vi "Load Configuration Database.vi"(8 "error in (no error)":errorcluster, 10 "Configuration Database Type":T1, 11 "Simulated Configuration Database in":refnum<class "Simulated Configuration Database.lvclass">) -> (0 "error out":errorcluster, 3 "Simulated Configuration Database out":refnum<class "Simulated Configuration Database.lvclass">)   [LabVIEW 2012, in "Simulated Configuration Database.lvlib" / "Simulated Configuration Database.lvclass"]
uses:
  Simulated Configuration Database.lvclass
  Configuration Database API/Configuration Database API/Configuration Type.ctl
  Configuration Database API/Configuration Database API/Record.ctl
  Configuration Database API/Configuration Database API/Configuration Database API.lvclass
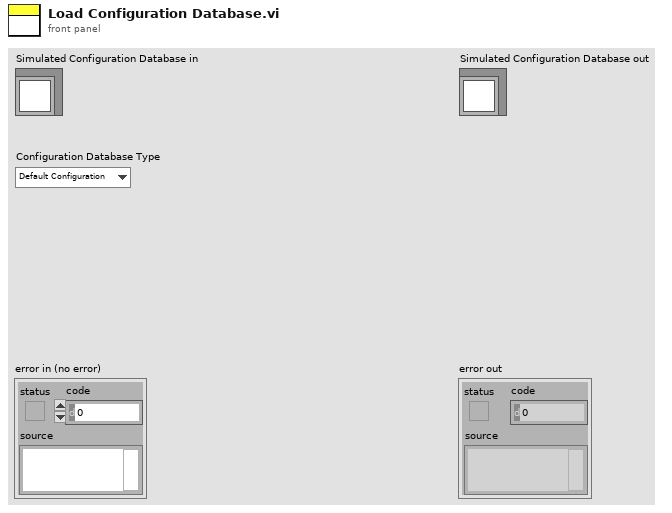
[diagram p1: front panel]
types:
  T1 = typedef "Configuration Database API.lvlib/Configuration Database API.lvclass/Configuration Type.ctl" = enum16{"Default Configuration", "Client Configuration"}
  T2 = typedef "Configuration Database API.lvlib/Configuration Database API.lvclass/Record.ctl" = cluster{"Wash Step":string, "Station":string, "Step Duration":u8}
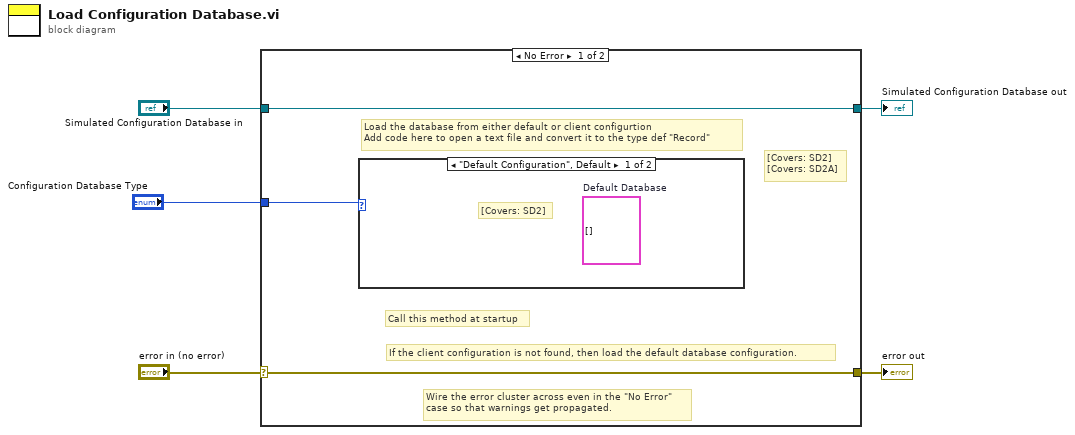
[diagram p0: block diagram]
diagram:
  n1 = case shown="No Error" "error in (no error)" {
    selector: "error in (no error)" -> [w7 w10]
    tunnel: [w7 w10] -> w4
    tunnel: [w8 w9] -> w2
    tunnel: "Simulated Configuration Database in" -> [w8 w9]
    tunnel: "Configuration Database Type" -> [w6 _]
    frame No Error {
      # "If the client configuration is not found, then load the default database configuration."
      # "Call this method at startup"
      # "[Covers: SD2]\n[Covers: SD2A]"
      # "Load the database from either default or client configurtion\nAdd code here to open a text file and convert it to the type def \"Record\""
      # "Wire the error cluster across even in the \"No Error\"\ncase so that warnings get propagated."
      n2 = case shown="\"Default Configuration\", Default" w6 {
        frame "Default Configuration", Default {
          (unwired) T2[] []  # Default Database
          # "[Covers: SD2]"
        }
        frame "Client Configuration" {
        }
      }
    }
    frame Error {
    }
  }
  "error out" <- w4
  "Simulated Configuration Database out" <- w2
